vi "Constants.vi"() -> ()   [LabVIEW 2018, in "UDP Shared.lvlib"]
doc: "Use this Global VI to access the GUIDs assigned to the page resources of the Custom Device."
uses:
  UDP Shared.lvlib
panel:
  in  "Tab Control":enum32{"GUIDS", "Constants", "Properties"}(tab)
  in  "UDP":string="39121477-5fba-42a1-80f3-109b32fabfd8"
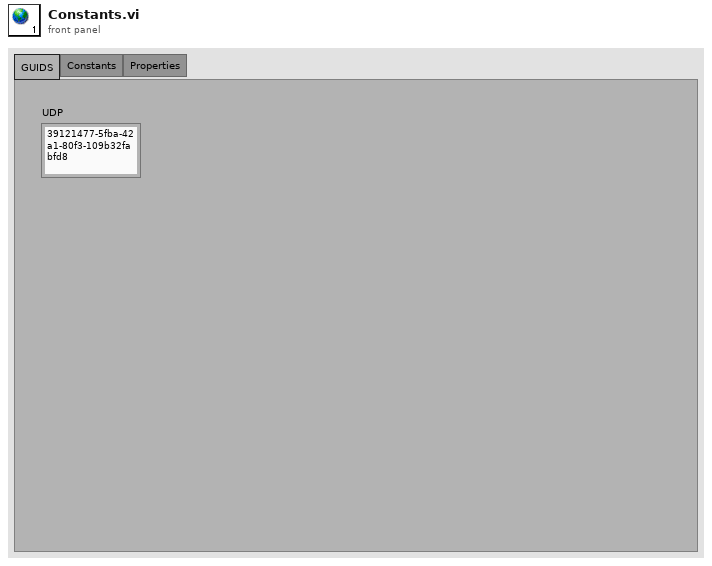
[diagram p1: front panel]
diagram:
